vi "test_Configure Response WaitSec.vi"(8 "error in (no error)":errorcluster, 11 "TestCase in":refnum<class "Instrument Addon Scripting API Messages Unit Tests.lvclass">) -> (0 "error out":errorcluster, 3 "TestCase out":refnum<class "Instrument Addon Scripting API Messages Unit Tests.lvclass">)   [LabVIEW 2019, in "Instrument Addon Scripting API Messages Unit Tests.lvclass"]
uses:
  Instrument Addon Scripting API Messages Unit Tests.lvclass
  Addon/Addon Shared/Types/FG Control.ctl
  APIs/Scripting API/TypeDefs/Wait Response Settings.ctl
  APIs/Scripting API/TypeDefs/Linked Channel.ctl
  <vilib>/NI VeriStand/Custom Device API/Custom Device Item Ref.ctl
  Addon/Addon Shared/Types/Response Parameters.ctl
  Addon/Addon Shared/Types/Linked Channel Cluster.ctl
  Addon/Addon Shared/Types/Response Wait Type.ctl
  Instrument Addon Scripting API Messages Unit Tests.lvclass/Instrument Addon Scripting API Messages Unit Tests.ctl
  Addon/Addon Shared/SubVIs/Constants.vi
  <vilib>/NI/NI VeriStand Advanced SysDef API/_SubVIs/SysDef.Search.GUID.vi
  <vilib>/NI VeriStand/Custom Device API/NI VeriStand - Get Item Property.vi
  <vilib>/NI VeriStand/Custom Device API/Get Item Property (String).vi
  <vilib>/NI VeriStand/Custom Device API/Get Item Property (String Array).vi
  <vilib>/NI VeriStand/Custom Device API/Get Item Property (Double).vi
  <vilib>/NI VeriStand/Custom Device API/Get Item Property (U32).vi
  <vilib>/NI VeriStand/Custom Device API/Get Item Property (Boolean).vi
  <vilib>/NI VeriStand/Custom Device API/NI VeriStand - Set Item Property.vi
  <vilib>/NI VeriStand/Custom Device API/Set Item Property (String).vi
  <vilib>/NI VeriStand/Custom Device API/Set Item Property (String Array).vi
  <vilib>/NI VeriStand/Custom Device API/Set Item Property (Double).vi
  <vilib>/NI VeriStand/Custom Device API/Set Item Property (U32).vi
  <vilib>/NI VeriStand/Custom Device API/Set Item Property (Boolean).vi
  APIs/Scripting API/Messages/Configure Response - Wait (sec).vi
  <vilib>/addons/_JKI Toolkits/VI Tester/TestCase.llb/TestCase.lvclass
  Instrument Addon Scripting API Test Assets/Instrument Addon Scripting API Test Assets.lvclass
  APIs/Scripting API/Instrument Addon Scripting API.lvlib
  <vilib>/NI VeriStand/Custom Device API/Custom Device API.lvlib
  Addon/Addon Shared/Instrument Addon Shared.lvlib
  <vilib>/NI/NI VeriStand Advanced SysDef API/SysDef API/Advanced System Definition.lvlib
  C:/Program Files (x86)/National Instruments/LabVIEW 2019/vi.lib/addons/_JKI Toolkits/VI Tester/TestCase.llb/TestCase.lvclass
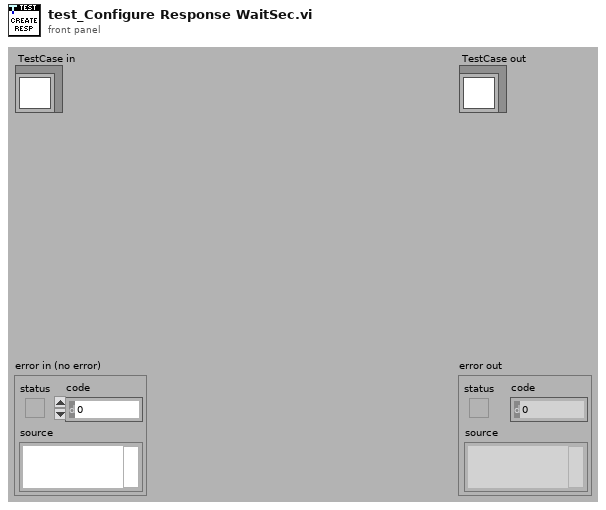
[diagram p1: front panel]
types:
  T1 = typedef "Instrument Addon Scripting API.lvlib/Wait Response Settings.ctl" = cluster{"Response Format":string, "Linked Channels":T2[], "Wait value (sec)":dbl, "Use Wait Channel":bool, "Channel Refnum":T3}
  T2 = typedef "Instrument Addon Scripting API.lvlib/Linked Channel.ctl" = cluster{"Variable Name":string, "Channel Refnum":T3}
  T3 = typedef "Custom Device API.lvlib/Custom Device Item Ref.ctl" = u64
  T4 = typedef "Instrument Addon Shared.lvlib/FG Control.ctl" = enum16{"Get", "Set"}
  T5 = typedef "Instrument Addon Shared.lvlib/Response Parameters.ctl" = cluster{"Response":string, "Linked Channels":T6[], "Type Value":dbl, "Wait Type":T7, "Use Channel":bool, "Channel Path":string}
  T6 = typedef "Instrument Addon Shared.lvlib/Linked Channel Cluster.ctl" = cluster{"Variable Name":string, "GUID":string}
  T7 = typedef "Instrument Addon Shared.lvlib/Response Wait Type.ctl" = enum16{"Byte Count", "Wait sec"}
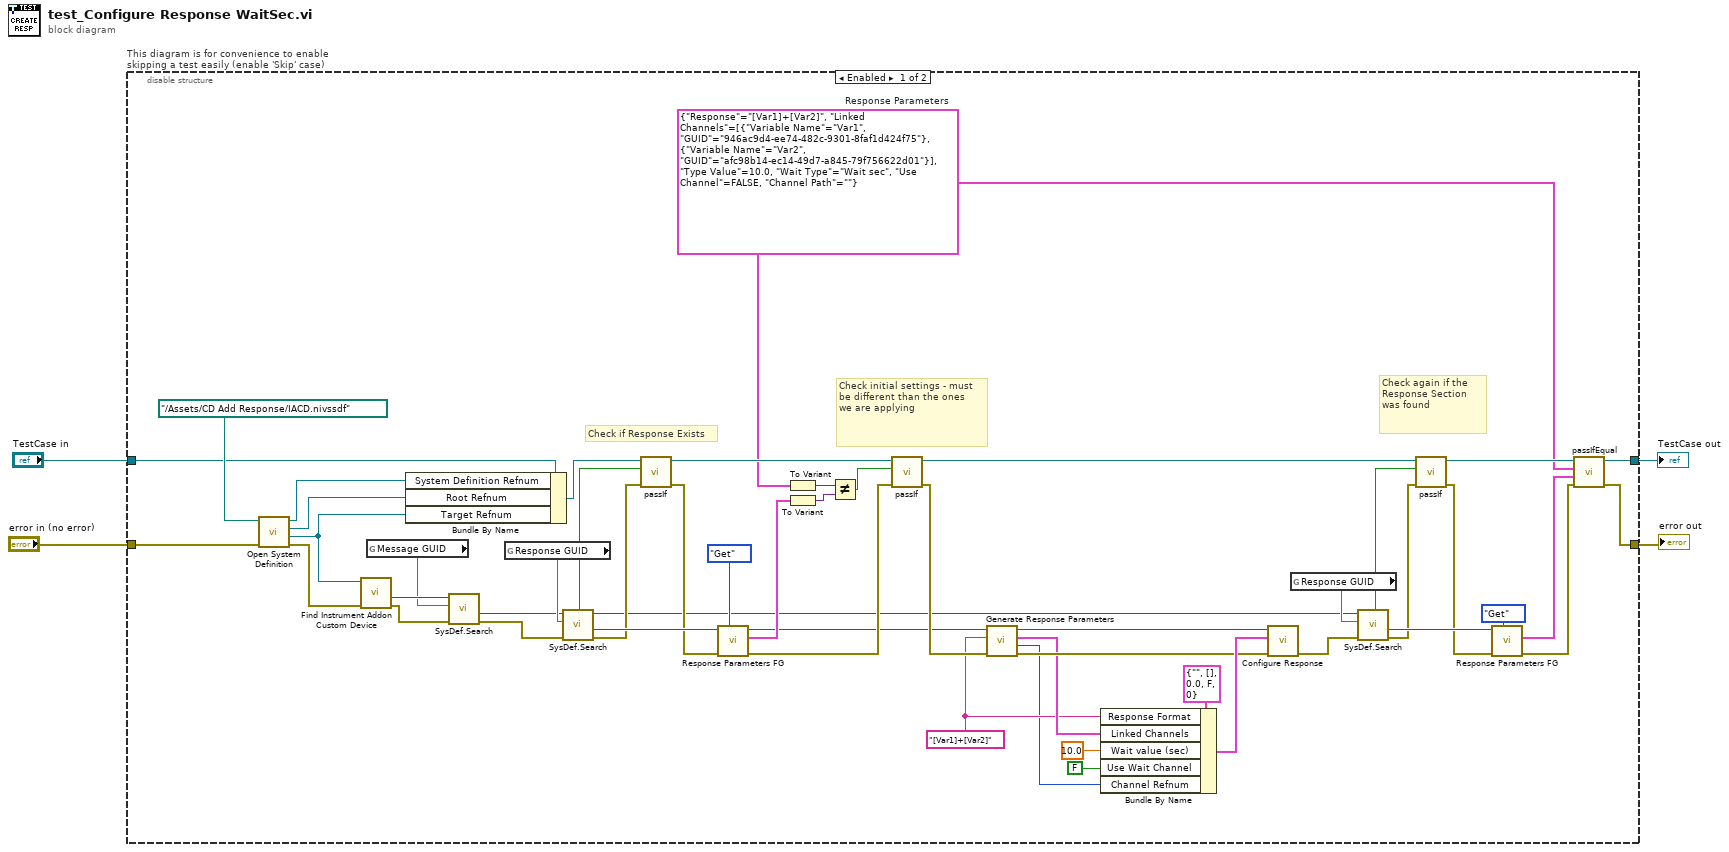
[diagram p0: block diagram]
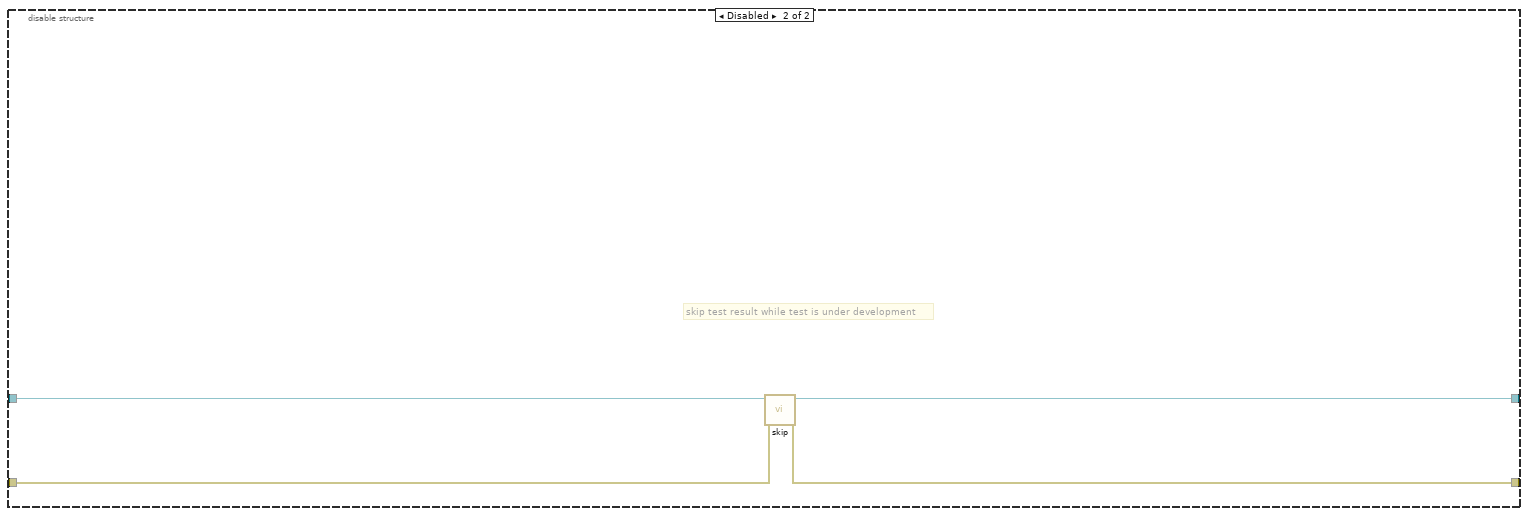
[diagram p2: hidden frame]
diagram:
  n1 = disable-structure "This diagram is for convenience to enable skipping a test easily (enable 'Skip' case)" shown="Enabled" {
    disable-tunnel: "TestCase in" -> [w12 w59]
    disable-tunnel: [w47 w57] -> w1
    disable-tunnel: [w46 w58] -> w3
    disable-tunnel: "error in (no error)" -> [w54 w56]
    frame Enabled {
      w19 = T5 {"Response"="[Var1]+[Var2]", "Linked Channels"=[{"Variable Name"="Var1", "GUID"="946ac9d4-ee74-482c-9301-8faf1d424f75"}, {"Variable Name"="Var2", "GUID"="afc98b14-ec14-49d7-a845-79f756622d01"}], "Type Value"=10.0, "Wait Type"=enum."Wait sec", "Use Channel"=FALSE, "Channel Path"=""}  # Response Parameters
      w14 = "[Var1]+[Var2]" ("Response Format")
      # "Check again if the Response Section was found"
      # "Check initial settings - must be different than the ones\nwe are applying"
      # "Check if Response Exists"
      n2 = call "Open System Definition.vi"("error in (no error)"=w54, "System Definition File"=path "../Assets/CD Add Response/IACD.nivssdf" ("SDF file")) -> ("error out"=w53:errorcluster, "Target Refnum"=w11:refnum<k24>, "Root Refnum"=w10:refnum<k24>, "System Definition Refnum"=w9:refnum<k24>)  [unwired: 6 in]
      n3 = call "Find Instrument Addon Custom Device.vi"("error in"=w53, "target in"=w11) -> ("error out"=w23:errorcluster, "NodeID"=w24:u64)  [unwired: 7 in, 1 out]
      n4 = global read "Constants.vi" "Message GUID"() -> (w22:string)
      n5 = Bundle By Name(cluster=w12, "System Definition Refnum"=w9, "Root Refnum"=w10, "Target Refnum"=w11) -> (w8:refnum<class "Instrument Addon Scripting API Messages Unit Tests.lvclass">)
      n6 = call-poly <vilib>:"SysDef.Search.vi"("error in (no error)"=w23, "GUID"=w22, "nodeID"=w24) -> ("error out"=w21:errorcluster, "Value out"=w20:u64)  [unwired: 5 in, 2 out]
      n7 = global read "Constants.vi" "Response GUID"() -> (w43:string)
      n8 = call-poly <vilib>:"SysDef.Search.vi"("error in (no error)"=w21, "GUID"=w43, "nodeID"=w20) -> ("error out"=w37:errorcluster, "Value out"=w44:u64, "nodeID out"=w5:u64, "Found?"=w38:bool)  [unwired: 5 in]
      n9 = call-dynamic "passIf.vi"("error in (no error)"=w37, "pass"=w38, "TestCase in"=w8) -> ("error out"=w36:errorcluster, "TestCase out"=w35:refnum<class "Instrument Addon Scripting API Messages Unit Tests.lvclass">)  [unwired: 7 in]
      n10 = call "Response Parameters FG.vi"("Action"=FG_Control."Get", "error in (no error)"=w36, "Item Ref in"=w44) -> ("error out"=w34:errorcluster, "Response Parameters"=w42:T5, "Item Ref out"=w16:T3)  [unwired: 6 in]
      n11 = To Variant(anything=w19) -> (Variant=w41:variant)
      n12 = To Variant(anything=w42) -> (Variant=w40:variant)
      n13 = Not Equal?(x=w41, y=w40) -> (x != y?=w39:bool)
      n14 = call-dynamic "passIf.vi"("error in (no error)"=w34, "pass"=w39, "TestCase in"=w35) -> ("error out"=w18:errorcluster, "TestCase out"=w33:refnum<class "Instrument Addon Scripting API Messages Unit Tests.lvclass">)  [unwired: 7 in]
      n15 = call "Generate Response Parameters.vi"("Error In"=w18, "Response String"=w14, "Response Channel in"=w16) -> ("Error Out"=w17:errorcluster, "Wait Channel Ref out"=w13:T3, "Linked Channels"=w15:T2[], "Response Channel out"=w6:T3)  [unwired: 5 in]
      n16 = Bundle By Name(cluster=T1 {"Response Format"="", "Linked Channels"=[], "Wait value (sec)"=0.0, "Use Wait Channel"=FALSE, "Channel Refnum"=0} ("Settings"), "Response Format"=w14, "Linked Channels"=w15, "Wait value (sec)"=10.0, "Use Wait Channel"=FALSE ("Use Byte Count channel"), "Channel Refnum"=w13) -> (w26:T1)
      n17 = call-poly "Configure Response.vi"("error in (no error)"=w17, "settings"=w26, "reponse refnum in"=w6) -> ("error out"=w49:errorcluster)  [unwired: 7 in, 1 out]
      n18 = global read "Constants.vi" "Response GUID"() -> (w50:string)
      n19 = call-poly <vilib>:"SysDef.Search.vi"("error in (no error)"=w49, "GUID"=w50, "nodeID"=w5) -> ("error out"=w32:errorcluster, "Value out"=w48:u64, "Found?"=w31:bool)  [unwired: 5 in, 1 out]
      n20 = call-dynamic "passIf.vi"("error in (no error)"=w32, "pass"=w31, "TestCase in"=w33) -> ("error out"=w30:errorcluster, "TestCase out"=w29:refnum<class "Instrument Addon Scripting API Messages Unit Tests.lvclass">)  [unwired: 7 in]
      n21 = call "Response Parameters FG.vi"("Action"=FG_Control."Get", "error in (no error)"=w30, "Item Ref in"=w48) -> ("error out"=w7:errorcluster, "Response Parameters"=w25:T5)  [unwired: 6 in, 1 out]
      n22 = call-dynamic "passIfEqual.vi"("error in (no error)"=w7, "y"=w25, "x"=w19, "TestCase in"=w29) -> ("error out"=w46:errorcluster, "TestCase out"=w47:refnum<class "Instrument Addon Scripting API Messages Unit Tests.lvclass">)  [unwired: 6 in]
    }
    frame Disabled {
      # "skip test result while test is under development"
      n23 = call <vilib>:"skip.vi"("error in (no error)"=w56, "TestCase in"=w59) -> ("error out"=w58:errorcluster, "TestCase out"=w57:refnum<class "Instrument Addon Scripting API Messages Unit Tests.lvclass">)  [unwired: 8 in]
    }
  }
  "error out" <- w3
  "TestCase out" <- w1
